vi "FormMain.vi"() -> ()   [LabVIEW 2012]
uses:
  S7Ref.vi
  resultShow.vi
panel:
  out "防错确认":bool
  out "rigStatus 2":string="提示信息"
  out "拾取控制器螺栓":bool
  out "拾取电机螺栓":bool
  in  "自动 2":bool
  out "拾取电机架螺栓":bool
  in  "控制器码":string
  in  "电机码":string
  in  "管柱码":string
  in  "countRight":u32
  in  "countLeft":u32
  out "三号气枪安装控制器支架":bool
  out "涂色标":bool=TRUE
  in  "判定设定 2":string[][](table)
  in  "参数设定 2":string[][](table)
  out "takesTime":string
  out "表格控件":string[][](table)
  out "FFT范围 2":string[][](table)
  out "管柱扫码":bool
  out "取电机胶垫":bool
  out "控制器扫码":bool
  out "涂色标":bool
  out "电机扫码":bool=TRUE
  out "一号气枪安装电机":bool
  out "输出扭矩":dbl caption="数值 24" format="%.1f Nm"
  in  "打开按钮":bool
  in  "自动":bool
  out "rigStatus":string="提示信息"
  out "connectionMode":string
  out "productsName":string
  out "userStatus":string
  out "userName":string
  out "放入工件":bool
  out "双手启动翻转":bool=TRUE
  out "双手启动翻转平位":bool
  out "二号气枪安装控制器":bool
  out "涂色标":bool
  out "取出工件":bool
  # "电机/控制器专配专机"
  # "广东和氏自动化技术股份有限公司"
  # "GUANGDONG HESH AUTOMATION TECHNOLOGY CO.,LTD."
  # "电机控制器安装步骤"
  # "控制器支架安装步骤"
  # "完成计数："
  # "完成计数："
  # "用时："
  # "："
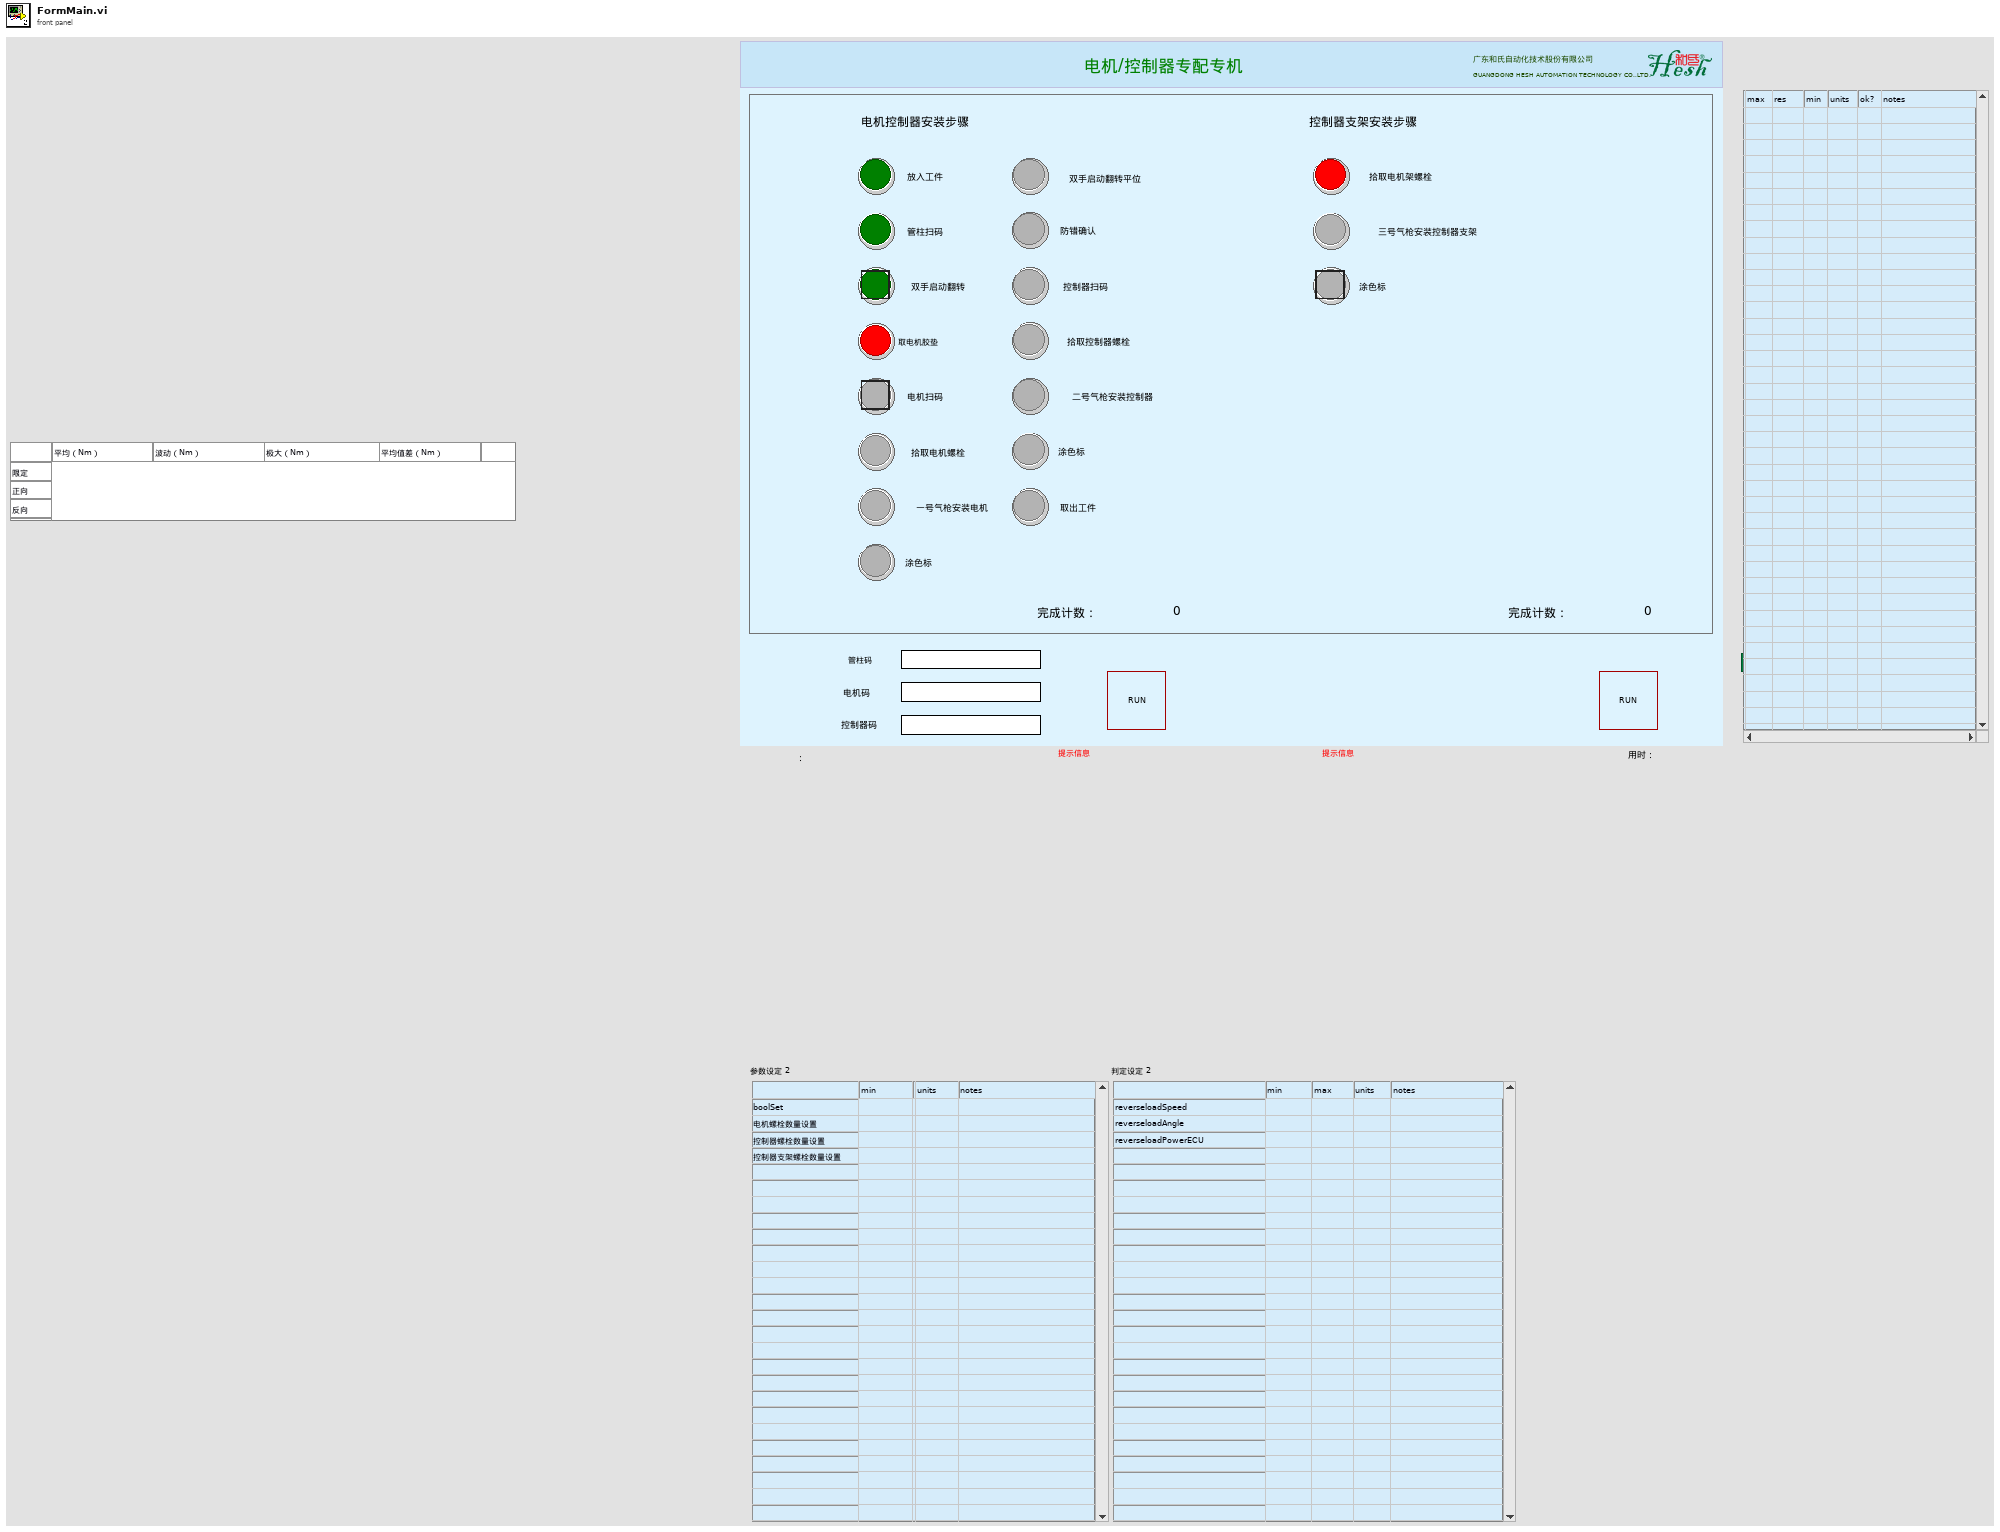
[diagram p1: front panel]
types:
  T1 = enum32{"Invalid", "Standard", "Closed", "Hidden", "Minimized", "Maximized"}
  T2 = cluster{"takesTime":refnum<vi>, "userStatus":refnum<vi>, "userName":refnum<vi>, "connectionMode":refnum<vi>, "productsName":refnum<vi>, "rigStatus":refnum<vi>, "管柱码":refnum<vi>, "电机码":refnum<vi>, "控制器码":refnum<vi>, "rigStatus 2":refnum<vi>}
  T3 = cluster{"userCode":string, "userName":string, "userStatus":string, "connectionMode":string, "takesTime":string, "countDone":string, "countOK":string, "countNG":string, "rigStatus":string, "productsName":string, "partCode1":string, "partCode2":string, "partCode3":string}
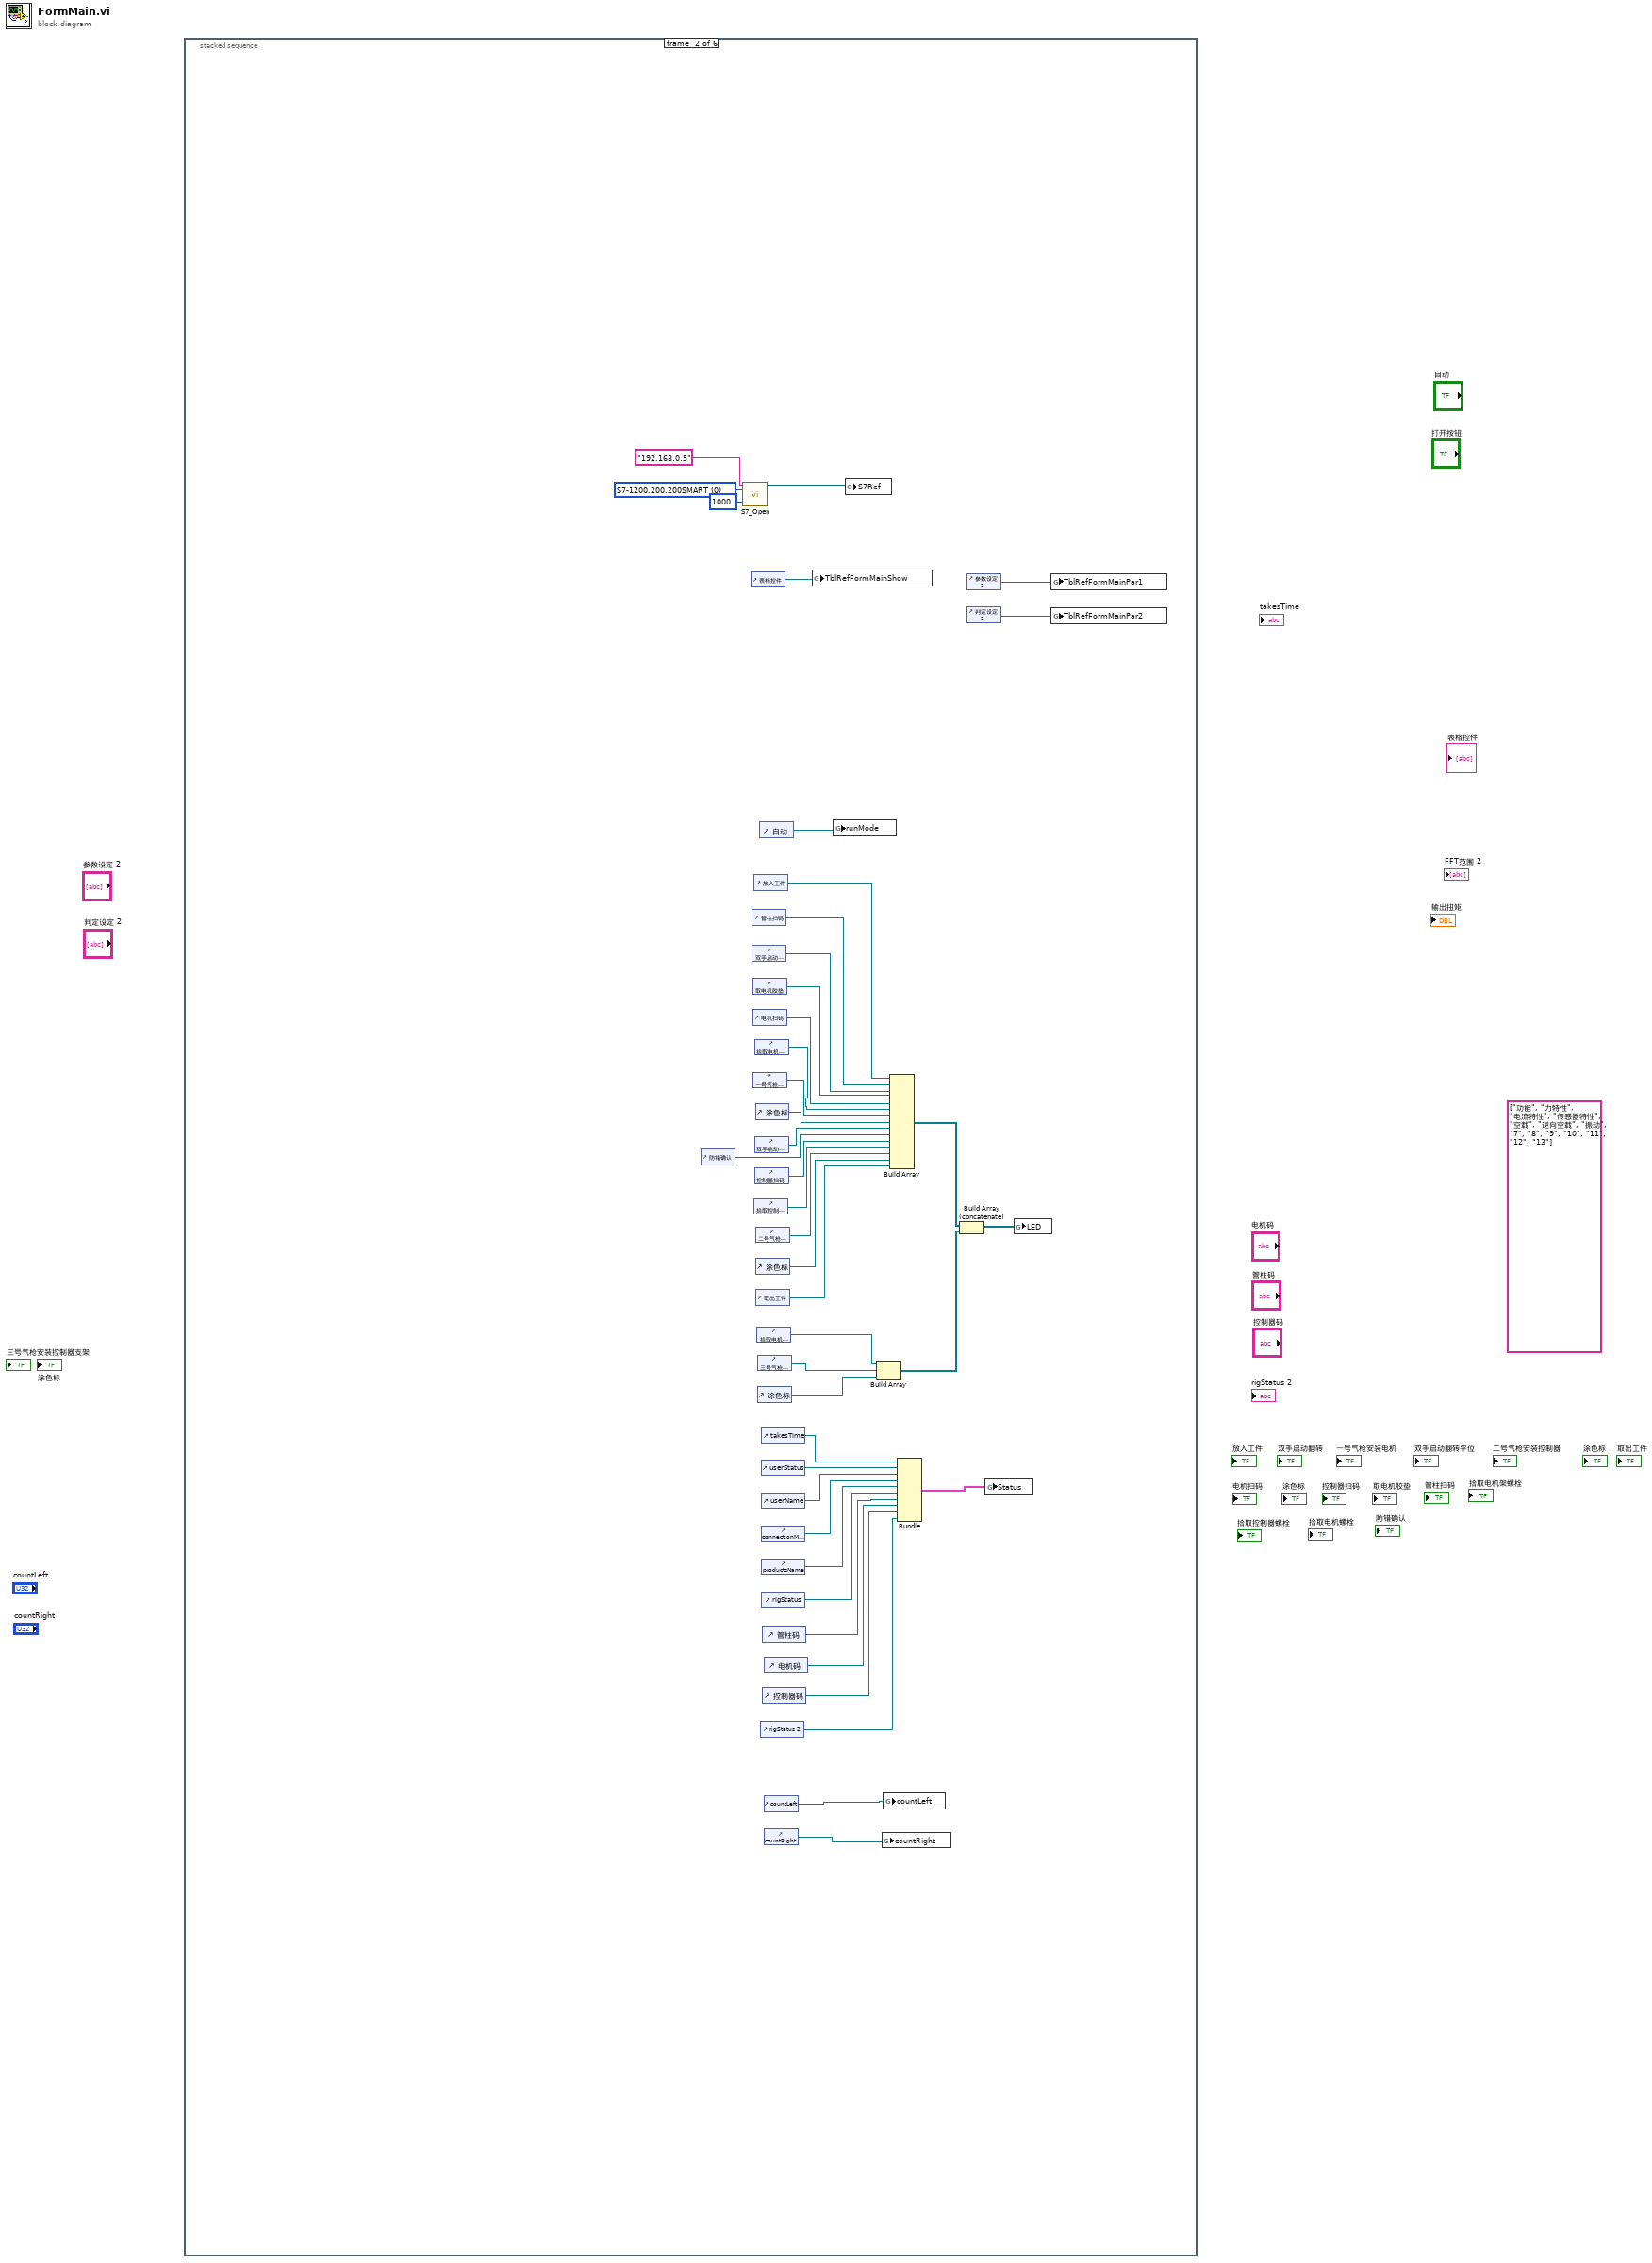
[diagram p0: block diagram]
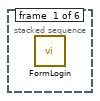
[diagram p2: hidden frame]
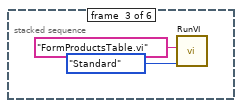
[diagram p3: hidden frame]
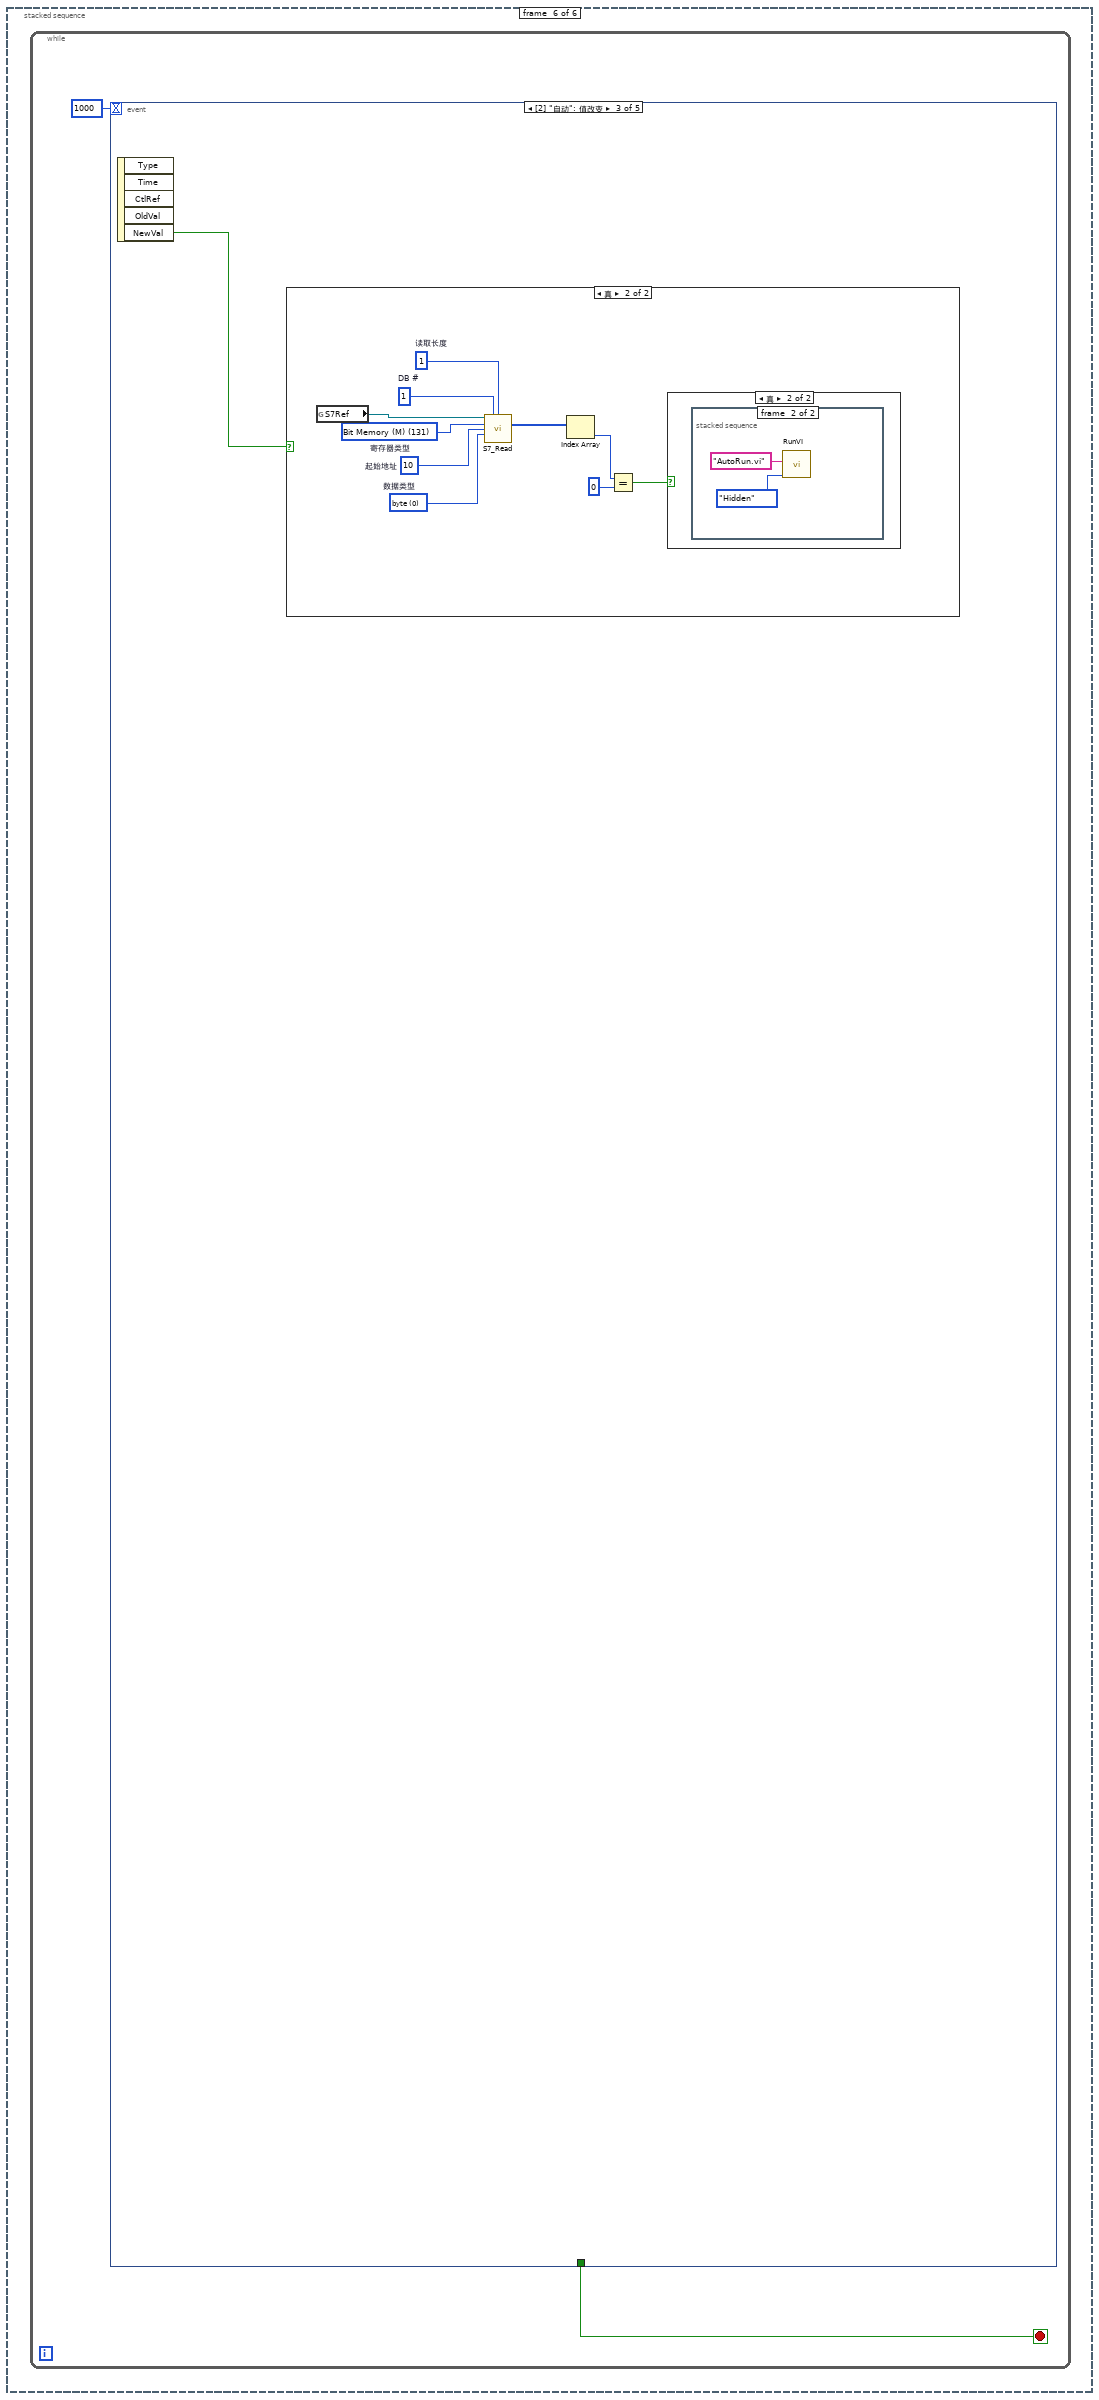
[diagram p6: hidden frame]
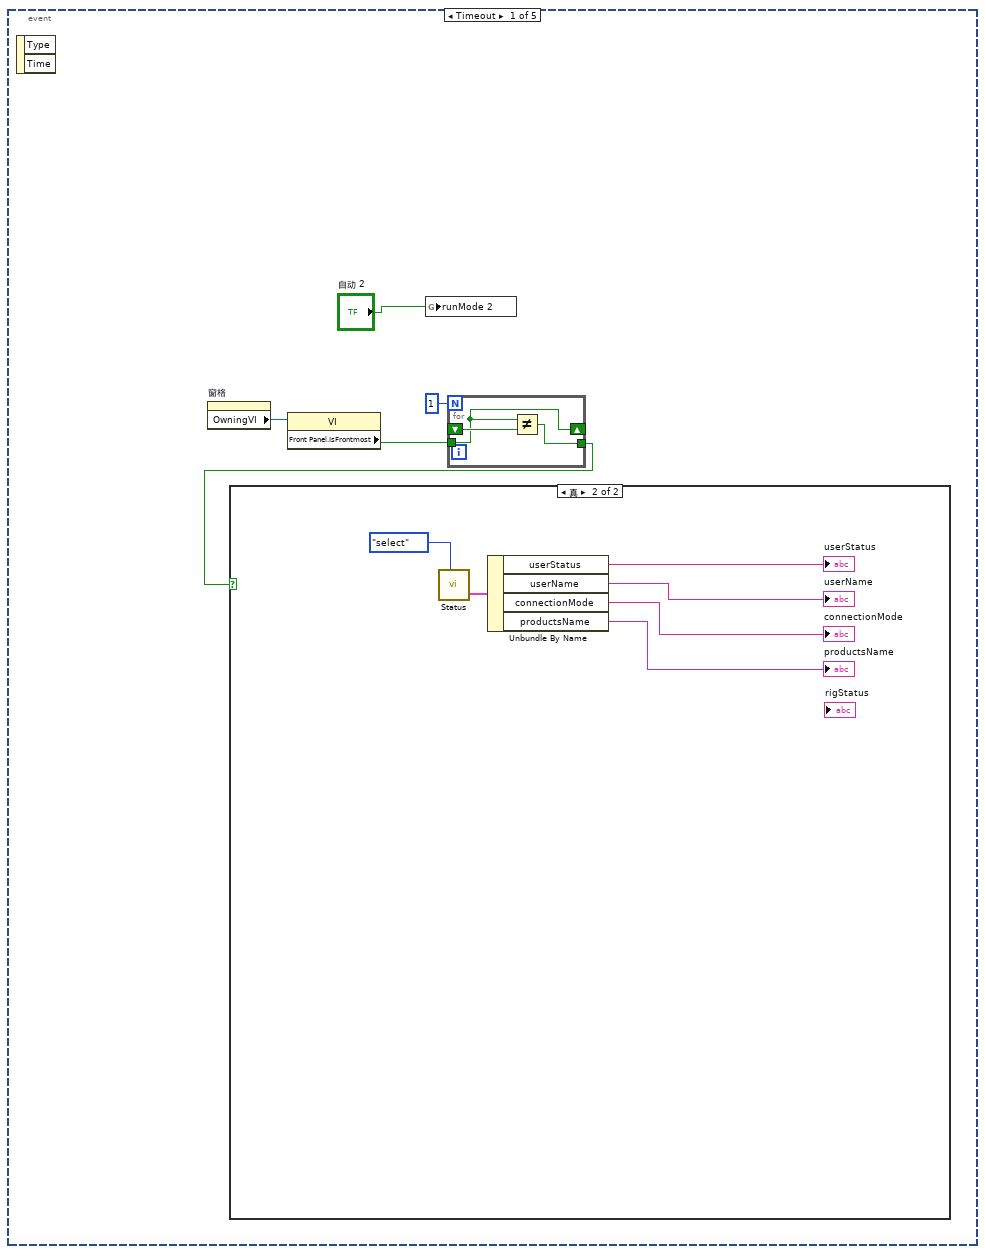
[diagram p7: hidden frame]
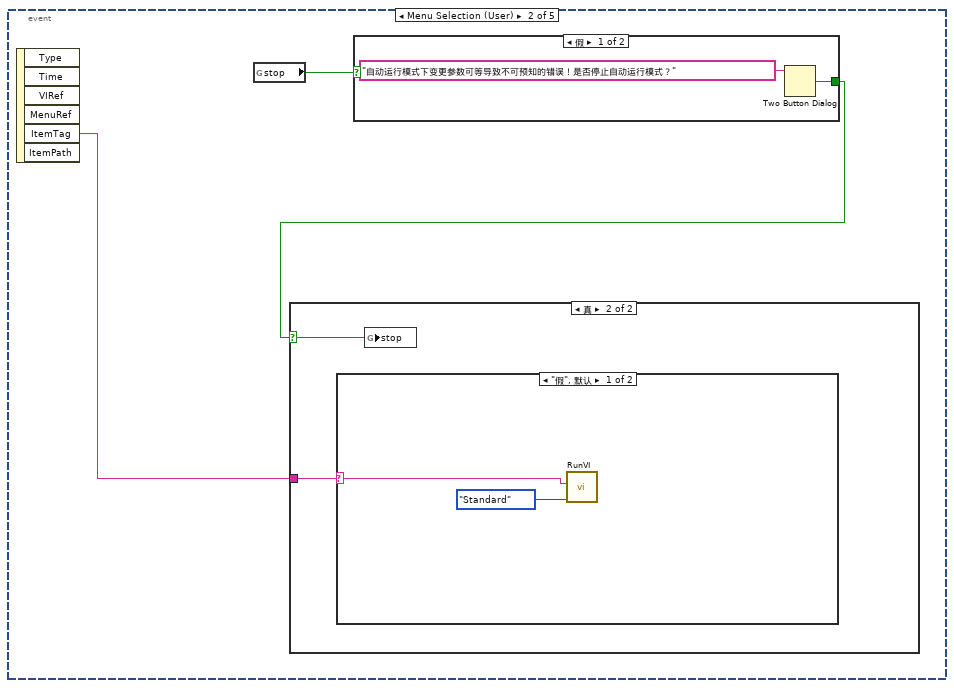
[diagram p9: hidden frame]
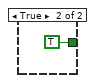
[diagram p10: hidden frame]
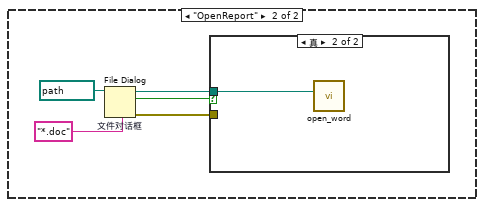
[diagram p12: hidden frame]
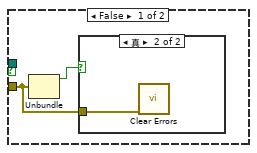
[diagram p13: hidden frame]
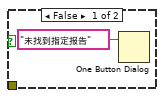
[diagram p14: hidden frame]
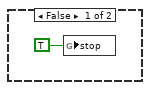
[diagram p15: hidden frame]
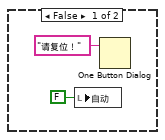
[diagram p16: hidden frame]
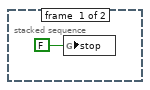
[diagram p17: hidden frame]
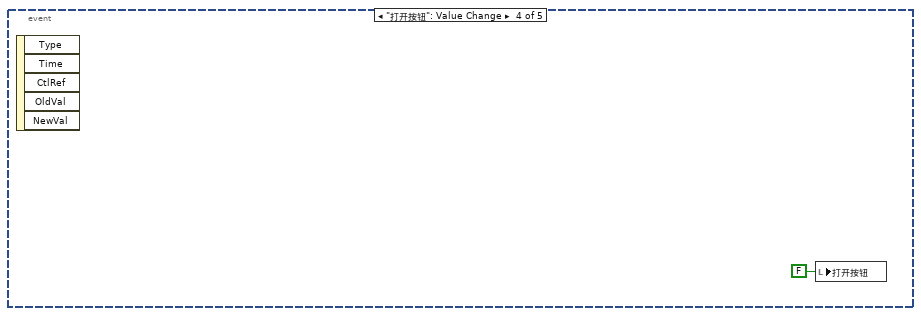
[diagram p18: hidden frame]
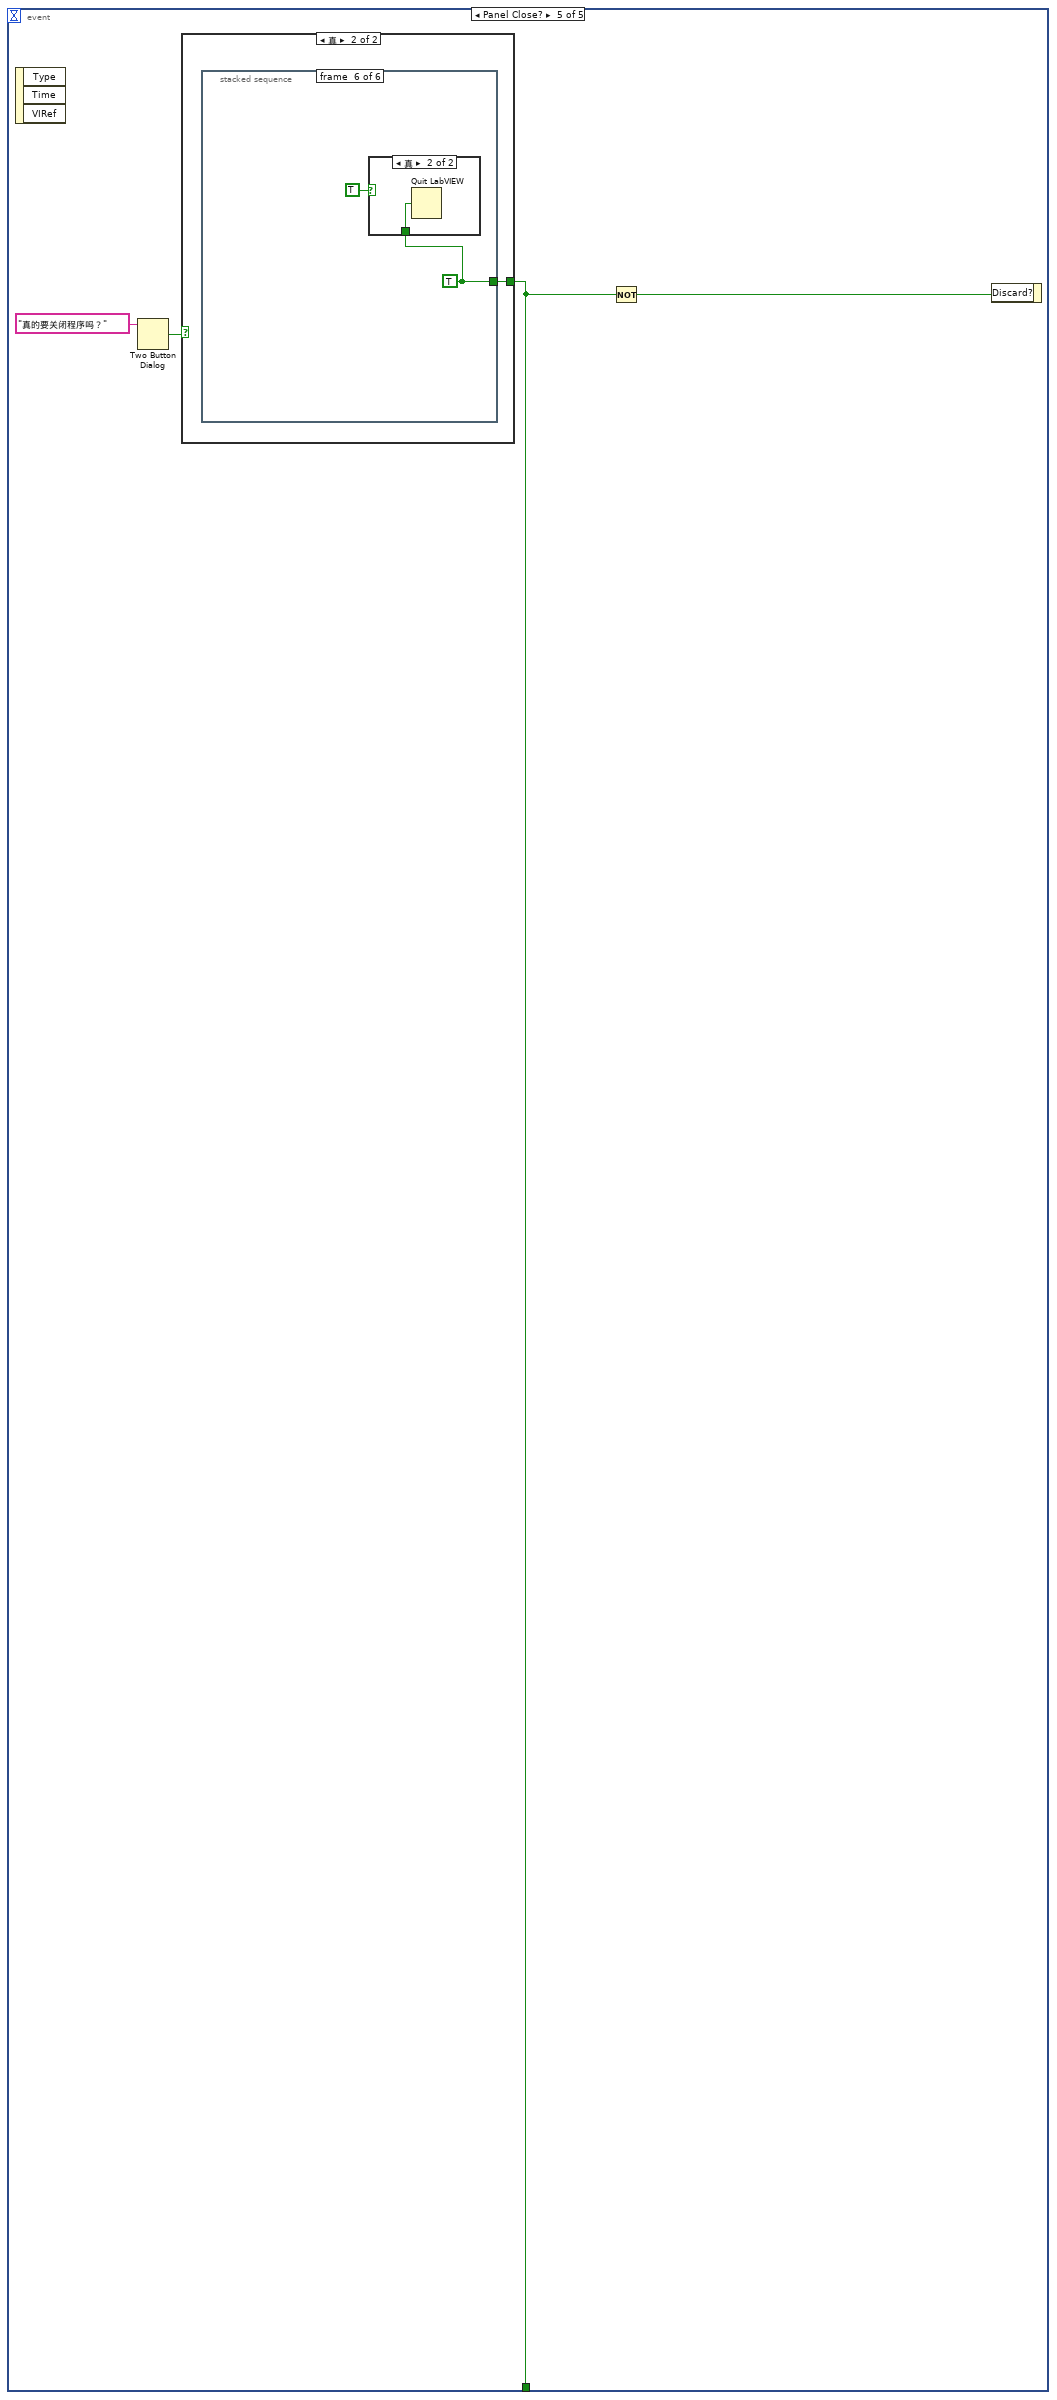
[diagram p19: hidden frame]
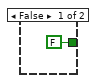
[diagram p20: hidden frame]
diagram:
  (unwired) string[] ["功能", "力特性", "电流特性", "传感器特性", "空载", "逆向空载", "振动", "7", "8", "9", "10", "11", "12", "13"] ("字符串[]")
  n1 = stacked-sequence {
    frame #0 {
      n2 = call "FormLogin.vi"() -> ()  [unwired: 12 in]
    }
    frame #1 {
      w40 = u8 0 items=["S7-1200.200.200SMART"=0, "S7-300"=2, "S7-400"=3] ("PLC 系列")
      n3 = control-ref of="防错确认"() -> (w1:refnum<vi>)
      n4 = call "S7_Open.vi"("IP 地址"="192.168.0.5", "PLC 系列"=w40, "超时（MS）"=1000) -> ("TCP"=w38:refnum<k5>)  [unwired: 10 in, 2 out]
      n5 = control-ref of="表格控件"() -> (w42:refnum<vi>)
      n6 = control-ref of="管柱扫码"() -> (w19:refnum<vi>)
      n7 = control-ref of="双手启动翻转"() -> (w18:refnum<vi>)
      n8 = control-ref of="取电机胶垫"() -> (w17:refnum<vi>)
      n9 = control-ref of="电机扫码"() -> (w16:refnum<vi>)
      n10 = control-ref of="一号气枪安装电机"() -> (w12:refnum<vi>)
      n11 = control-ref of="放入工件"() -> (w20:refnum<vi>)
      n12 = control-ref of="拾取控制器螺栓"() -> (w3:refnum<vi>)
      n13 = control-ref of="拾取电机螺栓"() -> (w8:refnum<vi>)
      n14 = control-ref of="双手启动翻转平位"() -> (w36:refnum<vi>)
      n15 = control-ref of="控制器扫码"() -> (w2:refnum<vi>)
      n16 = control-ref of="涂色标"() -> (w11:refnum<vi>)
      n17 = control-ref of="二号气枪安装控制器"() -> (w4:refnum<vi>)
      n18 = control-ref of="涂色标"() -> (w5:refnum<vi>)
      n19 = control-ref of="取出工件"() -> (w6:refnum<vi>)
      n20 = control-ref of="拾取电机架螺栓"() -> (w9:refnum<vi>)
      n21 = control-ref of="三号气枪安装控制器支架"() -> (w10:refnum<vi>)
      n22 = control-ref of="涂色标"() -> (w23:refnum<vi>)
      n23 = control-ref of="自动"() -> (w37:refnum<vi>)
      n24 = control-ref of="rigStatus 2"() -> (w7:refnum<vi>)
      n25 = control-ref of="takesTime"() -> (w29:refnum<vi>)
      n26 = control-ref of="userStatus"() -> (w35:refnum<vi>)
      n27 = control-ref of="userName"() -> (w34:refnum<vi>)
      n28 = control-ref of="connectionMode"() -> (w33:refnum<vi>)
      n29 = control-ref of="productsName"() -> (w32:refnum<vi>)
      n30 = control-ref of="rigStatus"() -> (w31:refnum<vi>)
      n31 = control-ref of="管柱码"() -> (w15:refnum<vi>)
      n32 = control-ref of="控制器码"() -> (w13:refnum<vi>)
      n33 = control-ref of="电机码"() -> (w14:refnum<vi>)
      n34 = control-ref of="countLeft"() -> (w22:refnum<vi>)
      n35 = control-ref of="countRight"() -> (w21:refnum<vi>)
      n36 = global write "resultShow.vi" "TblRefFormMainShow"(w42) -> ()
      n37 = global write "resultShow.vi" "runMode"(w37) -> ()
      n38 = global write "S7Ref.vi" "S7Ref"(w38) -> ()
      n39 = Build Array(w9, w10, w23) -> (w24:refnum<vi>[])
      n40 = global write "resultShow.vi" "countRight"(w21) -> ()
      n41 = global write "resultShow.vi" "countLeft"(w22) -> ()
      n42 = Build Array(w20, w19, w18, w17, w16, w8, w12, w11, w36, w1, w2, w3, w4, w5, w6) -> (w25:refnum<vi>[])
      n43 = Bundle("takesTime"=w29, "userStatus"=w35, "userName"=w34, "connectionMode"=w33, "productsName"=w32, "rigStatus"=w31, "管柱码"=w15, "电机码"=w14, "控制器码"=w13, "rigStatus 2"=w7) -> (w30:T2)  [unwired: 1 in]
      n44 = Build Array (concatenate)(w25, w24) -> (w26:refnum<vi>[])
      n45 = control-ref of="参数设定 2"() -> (w28:refnum<vi>)
      n46 = control-ref of="判定设定 2"() -> (w27:refnum<vi>)
      n47 = global write "resultShow.vi" "Status"(w30) -> ()
      n48 = global write "resultShow.vi" "LED"(w26) -> ()
      n49 = global write "resultShow.vi" "TblRefFormMainPar1"(w28) -> ()
      n50 = global write "resultShow.vi" "TblRefFormMainPar2"(w27) -> ()
    }
    frame #2 {
      n51 = call "RunVI.vi"("状态"=T1."Standard", "名称或相对路径"="FormProductsTable.vi") -> ()  [unwired: 9 in, 1 out]
    }
    frame #3 {
    }
    frame #4 {
    }
    frame #5 {
      n52 = while {
        stop <- w46 stop-if-true
        n53 = event shown="[2] \"自动\": 值改变" {
          selector: _ -> [_ _ _ _ _]
          dyn-events: _ -> [_ _ _ _ _]
          timeout: 1000 -> [_ _ _ _ _]
          tunnel: [_ _ _ _ w99] -> w46
          event Timeout {
            n54 = event-data() -> ()  [unwired: 1 in, 2 out]
            n55 = property on="窗格" class="Pane"() -> ("OwningVI"=w51:refnum<vi>)  [unwired: 2 in, 2 out]
            n56 = property class="VI"(reference=w51) -> ("Front Panel.IsFrontmost"=w49:bool)  [unwired: 1 in, 2 out]
            n57 = global write "resultShow.vi" "runMode 2"("自动 2") -> ()
            n58 = for {
              N: 1 -> [_]
              shift-right: [w59] -> _
              shift-left: _ -> [w60]
              tunnel: w49 -> [w59]
              tunnel: [w58] -> w48
              n59 = Not Equal?(x=w59, y=w60) -> (x != y?=w58:bool)
            }
            n60 = case shown="真" w48 {
              frame False {
              }
              frame True {
                n61 = call "Status.vi"("模式"=enum16{"select", "insert", "update", "delete"}."select") -> ("元素"=w56:T3)  [unwired: 10 in]
                n62 = Unbundle By Name(w56) -> ("userStatus"=→"userStatus":string, "userName"=→"userName":string, "connectionMode"=→"connectionMode":string, "productsName"=→"productsName":string)
              }
            }
          }
          event Menu Selection (User) {
            n63 = event-data() -> ("ItemTag"=w63:string)  [unwired: 1 in, 5 out]
            n64 = global read "全局 3.vi" "stop"() -> (w62:bool)
            n65 = case shown="假" w62 {
              tunnel: [w64 TRUE ("T button?")] -> w61
              frame False {
                n66 = Two Button Dialog(message="自动运行模式下变更参数可等导致不可预知的错误！是否停止自动运行模式？" ("消息")) -> (T button?=w64:bool)  [unwired: 2 in]
              }
              frame True {
              }
            }
            n67 = case shown="真" w61 {
              selector: w61 -> [_ w67]
              tunnel: w63 -> [_ w68]
              frame False {
              }
              frame True {
                n68 = case shown="\"假\", 默认" w68 {
                  selector: w68 -> [w69 _]
                  frame "假", Default {
                    n69 = call "RunVI.vi"("状态"=T1."Standard", "名称或相对路径"=w69) -> ()  [unwired: 9 in, 1 out]
                  }
                  frame "OpenReport" {
                    n70 = File Dialog "文件对话框"(6:"*.doc" ("prompt"), 11:path "D:/报表" ("开始路径")) -> (0:w71:errorcluster, 2:w73:bool, 3:w72:path)  [unwired: 1 in, 5 out]
                    n71 = case shown="真" w73 {
                      tunnel: w72 -> [_ w80]
                      tunnel: w71 -> [w76 _]
                      frame False {
                        n72 = Unbundle(w76) -> ("status"=w77:bool)  [unwired: 2 out]
                        n73 = case shown="真" w77 {
                          tunnel: w76 -> [_ w79]
                          frame False {
                            n74 = One Button Dialog(message="未找到指定报告" ("消息")) -> ()  [unwired: 1 in, 1 out]
                          }
                          frame True {
                            n75 = call <vilib>:"Clear Errors.vi"("error in (no error)"=w79) -> ()  [unwired: 6 in, 1 out]
                          }
                        }
                      }
                      frame True {
                        n76 = call "open_word.vi"("所选路径"=w80) -> ()  [unwired: 11 in]
                      }
                    }
                  }
                }
                n77 = global write "全局 3.vi" "stop"(w67) -> ()
              }
            }
          }
          event "自动": Value Change {
            n78 = event-data() -> ("NewVal"=w81:bool)  [unwired: 1 in, 4 out]
            n79 = case shown="真" w81 {
              frame False {
                n80 = global write "全局 3.vi" "stop"(TRUE ("布尔 1")) -> ()
              }
              frame True {
                w86 = u32 10  # 起始地址
                w88 = u16 0 items=["byte", "word", "Dword"]  # 数据类型
                w89 = u8 131 items=["I/O (P)"=128, "Input (I)"=129, "Output (Q)"=130, "Bit Memory (M)"=131, "Data (DB)"=132, "Instance Data (DI)"=133, "Local Data (L)"=134, "Predecessor Local Data (VL)"=135]  # 寄存器类型
                w90 = u16 1  # 读取长度
                w91 = u16 1  # DB #
                n81 = global read "S7Ref.vi" "S7Ref"() -> (w92:refnum<k5>)
                n82 = call "S7_Read.vi"("TCP"=w92, "DB #"=w91, "读取长度"=w90, "寄存器类型"=w89, "起始地址"=w86, "数据类型"=w88) -> ("数据"=w87:u32[])  [unwired: 6 in, 3 out]
                n83 = Index Array(array=w87) -> (element=w85:u32)  [unwired: 1 in]
                n84 = Equal?(x=w85, y=u32 0) -> (x = y?=w83:bool)
                n85 = case shown="真" w83 {
                  frame False {
                    n86 = local write "自动"(FALSE ("自动")) -> ()
                    n87 = One Button Dialog(message="请复位！" ("消息")) -> ()  [unwired: 1 in, 1 out]
                  }
                  frame True {
                    n88 = stacked-sequence {
                      frame #0 {
                        n89 = global write "全局 3.vi" "stop"(FALSE ("布尔 1")) -> ()
                      }
                      frame #1 {
                        n90 = call "RunVI.vi"("状态"=T1."Hidden", "名称或相对路径"="AutoRun.vi") -> ()  [unwired: 9 in, 1 out]
                      }
                    }
                  }
                }
              }
            }
          }
          event "打开按钮": Value Change {
            n91 = event-data() -> ()  [unwired: 1 in, 5 out]
            n92 = local write "打开按钮"(FALSE ("打开按钮")) -> ()
          }
          event Panel Close? {
            n93 = event-data() -> ()  [unwired: 1 in, 3 out]
            n94 = Two Button Dialog(message="真的要关闭程序吗？" ("消息")) -> (T button?=w100:bool)  [unwired: 2 in]
            n95 = case shown="真" w100 {
              tunnel: [FALSE w104] -> w99
              frame False {
              }
              frame True {
                n96 = stacked-sequence {
                  tunnel: [_ _ _ _ _ w112] -> w104
                  frame #0 {
                    n97 = for {
                      tunnel: string[] ["AutoRun.vi", "FormCamera.vi"] -> [w106] mode=indexing
                      n98 = call "CloseVI.vi"("名称或相对路径"=w106) -> ()  [unwired: 10 in, 1 out]
                    }
                  }
                  frame #1 {
                    n99 = shared-variable ".\\共享变量.lvlib\\string_5"("关闭程序中" ("string_5")) -> ()  [unwired: 1 in, 1 out]
                    n100 = global write "全局 3.vi" "stop"(TRUE ("布尔 2")) -> ()
                  }
                  frame #2 {
                    n101 = Wait (ms)(milliseconds to wait=u32 500 ("等待时间（毫秒）")) -> ()  [unwired: 1 out]
                  }
                  frame #3 {
                  }
                  frame #4 {
                    n102 = global read "S7Ref.vi" "S7Ref"() -> (w110:refnum<k5>)
                    n103 = call "S7_Close.vi"("TCP Connection Ref"=w110) -> ()  [unwired: 10 in, 1 out]
                  }
                  frame #5 {
                    w112 = TRUE
                    n104 = case shown="真" TRUE {
                      tunnel: w112 -> [_ w113]
                      frame False {
                      }
                      frame True {
                        n105 = Quit LabVIEW(quit? (T)=w113) -> ()
                      }
                    }
                  }
                }
              }
            }
            n106 = Not(x=w99) -> (.not. x?=w101:bool)
            n107 = event-data("Discard?"=w101) -> ()  [unwired: 1 in, 1 out]
          }
        }
      }
    }
  }
